vi "Save Restore Script.vi"(5 "Script Name":string, 6 "File Path":string, 7 "Script Variable":string, 8 "error in (no error)":errorcluster, 9 "Memory Type (0: Nonvolatile Memory)":i32(ring) items=["Nonvolatile Memory ", "USB Flash Drive"], 10 "Operation (0: Save)":i32(ring) items=["Save", "Restore"], 11 "VISA resource name":refnum<visa-resource-name>) -> (0 "error out":errorcluster, 3 "VISA resource name out":refnum<visa-resource-name>)   [LabVIEW 2017, in "Keithley 2600 Series.lvlib"]
doc: "Saves or restores a script."
uses:
  <instrlib>/Keithley 2600 Series/Keithley 2600 Series.lvlib
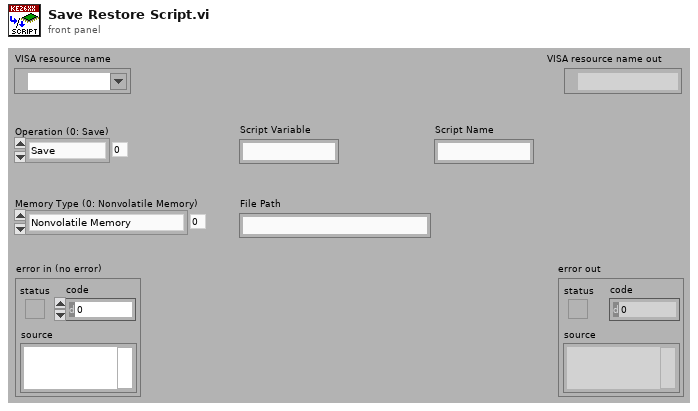
[diagram p1: front panel]
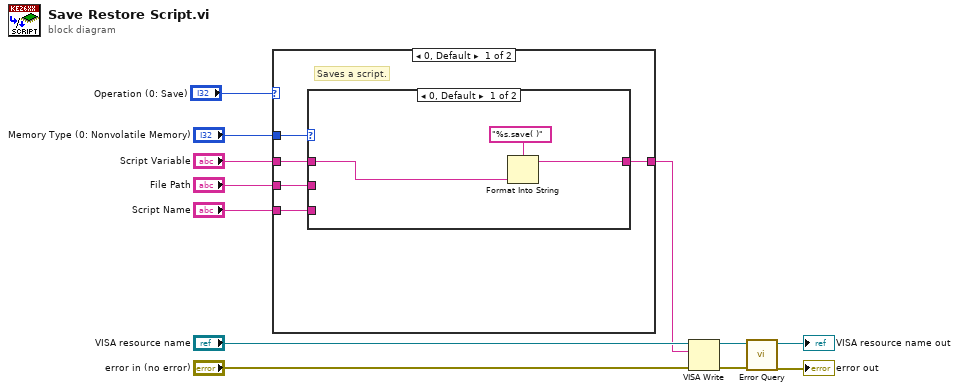
[diagram p0: block diagram]
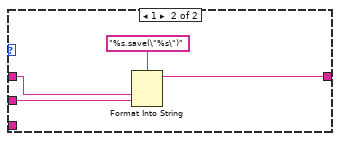
[diagram p2: hidden frame]
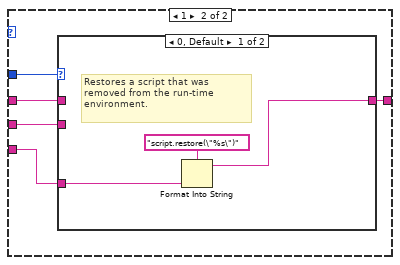
[diagram p3: hidden frame]
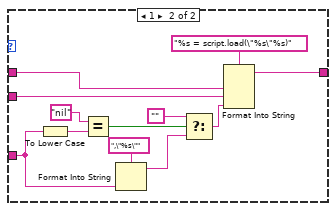
[diagram p4: hidden frame]
diagram:
  n1 = case shown="0, Default" "Operation (0: Save)" {
    tunnel: "Memory Type (0: Nonvolatile Memory)" -> [w14 w29]
    tunnel: "Script Name" -> [w15 w28]
    tunnel: [w17 w27] -> w4
    tunnel: "Script Variable" -> [w16 w26]
    tunnel: "File Path" -> [w13 w25]
    frame 0, Default {
      # "Saves a script."
      n2 = case shown="0, Default" w14 {
        tunnel: [w19 w23] -> w17
        tunnel: w16 -> [w18 w22]
        tunnel: w15 -> [_ _]
        tunnel: w13 -> [_ w21]
        frame 0, Default {
          n3 = Format Into String(format string="%s.save( )", w18) -> (resulting string=w19:string)  [unwired: 2 in, 1 out]
        }
        frame 1 {
          n4 = Format Into String(format string="%s.save(\"%s\")", w22, w21) -> (resulting string=w23:string)  [unwired: 2 in, 1 out]
        }
      }
    }
    frame 1 {
      n5 = case shown="0, Default" w29 {
        tunnel: w28 -> [w31 w33]
        tunnel: [w30 w42] -> w27
        tunnel: w26 -> [_ w43]
        tunnel: w25 -> [_ w41]
        frame 0, Default {
          # "Restores a script that was removed from the run-time environment."
          n6 = Format Into String(format string="script.restore(\"%s\")", w31) -> (resulting string=w30:string)  [unwired: 2 in, 1 out]
        }
        frame 1 {
          n7 = To Lower Case(string=w33) -> (all lower case string=w34:string)
          n8 = Equal?(x="nil" ("y"), y=w34) -> (x = y?=w39:bool)
          n9 = Format Into String(format string=",\"%s\"", w33) -> (resulting string=w40:string)  [unwired: 2 in, 1 out]
          n10 = Select(t="", s=w39, f=w40) -> (s? t:f=w36:string)
          n11 = Format Into String(format string="%s = script.load(\"%s\"%s)", w43, w41, w36) -> (resulting string=w42:string)  [unwired: 2 in, 1 out]
        }
      }
    }
  }
  n12 = VISA Write(VISA resource name="VISA resource name", write buffer=w4, error in (no error)="error in (no error)") -> (VISA resource name out=w10:refnum<visa-resource-name>, error out=w9:errorcluster)  [unwired: 1 out]
  n13 = call <instrlib>:"Error Query.vi"("error in (no error)"=w9, "VISA resource name"=w10) -> ("error out"=→"error out":errorcluster, "VISA resource name out"=→"VISA resource name out":refnum<visa-resource-name>)  [unwired: 6 in, 2 out]
